vi "ErrorIfInitialized.vi"(8 "error in (no error)":errorcluster, 11 "IAmGLF in":refnum<class "IAmGLF.lvclass">) -> (0 "error out":errorcluster, 3 "IAmGLF out":refnum<class "IAmGLF.lvclass">)   [LabVIEW 2020, in "GLF.lvlib" / "IAmGLF.lvclass"]
uses:
  IAmGLF.lvclass
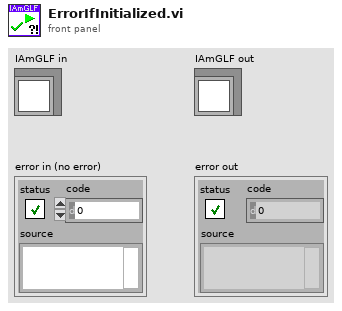
[diagram p1: front panel]
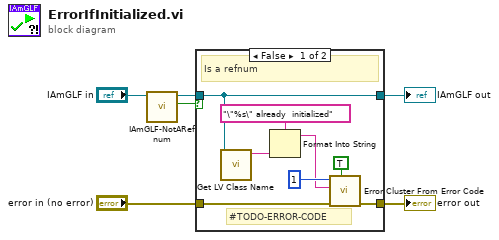
[diagram p0: block diagram]
diagram:
  n1 = call-dynamic "IAmGLF-NotARefnum.vi"("IAmGLF in"="IAmGLF in") -> ("Not A Valid Refnum?"=w6:bool, "IAmGLF out"=w1:refnum<class "IAmGLF.lvclass">)  [unwired: 9 in]
  n2 = case shown="False" w6 {
    tunnel: "error in (no error)" -> [w10 w16]
    tunnel: [w14 w16] -> w3
    tunnel: [w11 w15] -> w2
    tunnel: w1 -> [w11 w15]
    frame False {
      # "#TODO-ERROR-CODE"
      # "Is a refnum"
      n3 = call <vilib>:"Get LV Class Name.vi"("object"=w11) -> ("class name"=w8:string)  [unwired: 9 in, 1 out]
      n4 = Format Into String(format string="\"%s\" already  initialized" ("error message (\"\")"), w8) -> (resulting string=w9:string)  [unwired: 2 in, 1 out]
      n5 = call <vilib>:"Error Cluster From Error Code.vi"("show call chain? (False)"=TRUE, "error in (no error)"=w10, "error message (\"\")"=w9, "error code (0)"=1) -> ("error out"=w14:errorcluster)  [unwired: 5 in]
    }
    frame True {
      # "Not a refnum"
    }
  }
  "error out" <- w3
  "IAmGLF out" <- w2
